vi "Add New Object.vi"(7 "NewObject in":refnum<vi>, 8 "error in (no error)":errorcluster, 9 "Translation":T1, 10 "Color":u32(colorbox), 11 "Scene: Object":refnum<vi>) -> (0 "error out":errorcluster, 3 "SceneObject out":refnum<vi>)   [LabVIEW 2013]
doc: "This VI allows to add a new 3D object to a 3D object and set his position and his color."
uses:
  <vilib>/Utility/miscctls.llb/LV3DPointTypeDef.ctl
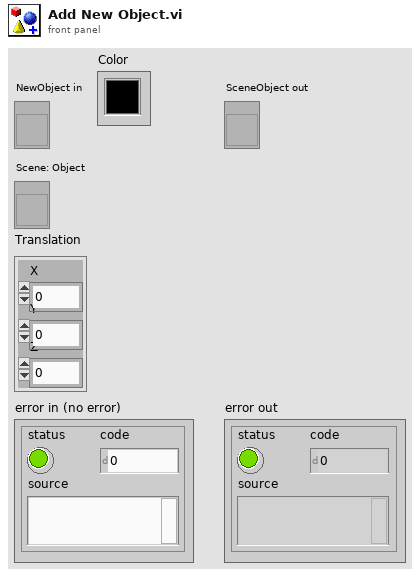
[diagram p1: front panel]
types:
  T1 = typedef "LV3DPointTypeDef.ctl" = cluster{"X":sgl, "Y":sgl, "Z":sgl}
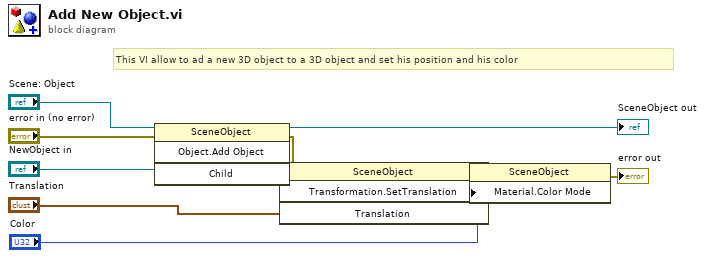
[diagram p0: block diagram]
diagram:
  # "This VI allow to ad a new 3D object to a 3D object and set his position and his color"
  n1 = invoke class="SceneObject" method="Object.Add Object"(reference="Scene: Object", error in="error in (no error)", "Child"="NewObject in") -> (reference out=→"SceneObject out":refnum<vi>, error out=w11:errorcluster, "Child"=w9:refnum<vi>)  [unwired: 1 in, 1 out]
  n2 = invoke class="SceneObject" method="Transformation.SetTranslation"(reference=w9, error in=w11, "Translation"="Translation") -> (reference out=w3:refnum<vi>, error out=w4:errorcluster)  [unwired: 1 in, 2 out]
  n3 = property class="SceneObject"(reference=w3, error in=w4, "Material.Color Mode"="Color") -> (error out=→"error out":errorcluster)  [unwired: 1 out]
